vi "05-调用dotnetdll.vi"() -> ()   [LabVIEW 2015]
uses:
  Interop.TSMasterAPI.dll
panel:
  in  "AChn":i32(ring) items=["CHN1", "CHN2", "CHN3", "CHN4", "CHN5", "CHN6", "CHN7", "CHN8", "CHN9", "CHN10", "CHN11", "CHN12", "CHN13", "CHN14", "CHN15", "CHN16", "CHN17", "CHN18", "CHN19", "CHN20", "CHN21", "CHN22", "CHN23", "CHN24", "CHN25", "CHN26", "CHN27", "CHN28", "CHN29", "CHN30", "CHN31", "CHN32"]
  in  "size":i32
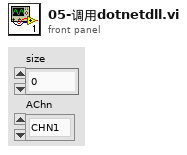
[diagram p1: front panel]
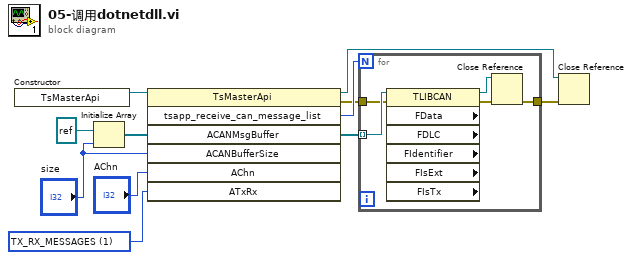
[diagram p0: block diagram]
diagram:
  w6 = u8 1 items=["ONLY_RX_MESSAGES", "TX_RX_MESSAGES"] ("ATxRx")
  n1 = constructor class="TsMasterApi"() -> (reference out=w11:refnum<k24>)  [unwired: 3 in, 2 out]
  n2 = Initialize Array(refnum<k24> refnum, "size") -> (w9:refnum<k24>[])
  n3 = invoke on="调用节点" class="TsMasterApi" method="tsapp_receive_can_message_list"(reference=w11, "ACANMsgBuffer"=w9, "ACANBufferSize"="size", "AChn"="AChn", "ATxRx"=w6) -> (reference out=w3:refnum<k24>, error out=w1:errorcluster, "tsapp_receive_can_message_list"=w5:i32, "ACANMsgBuffer"=w4:refnum<k24>[])  [unwired: 2 in, 3 out]
  n4 = for {
    N: w5 -> [_]
    tunnel: w4 -> [w16] mode=indexing
    tunnel: [w14] -> w2
    tunnel: w1 -> [w12]
    n5 = property on="属性节点" class="TLIBCAN" props=["FData", "FDLC", "FIdentifier", "FIsExt", "FIsTx"](reference=w16, error in=w12) -> (reference out=w15:refnum<k24>, error out=w13:errorcluster)  [unwired: 5 out]
    n6 = Close Reference(reference=w15, error in (no error)=w13) -> (error out=w14:errorcluster)
  }
  n7 = Close Reference(reference=w3, error in (no error)=w2) -> ()  [unwired: 1 out]
